vi "4.vi"() -> ()   [LabVIEW 2017]
panel:
  out "XY图":cluster{dbl[], dbl[]}[](graph)
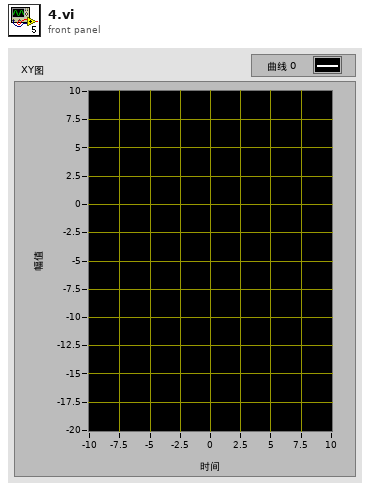
[diagram p1: front panel]
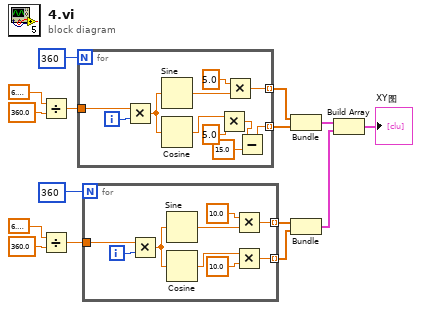
[diagram p0: block diagram]
diagram:
  n1 = Divide(x=6.283185307179586, y=360.0) -> (x/y=w12:dbl)
  n2 = Divide(x=6.283185307179586, y=360.0) -> (x/y=w6:dbl)
  n3 = for {
    N: 360 -> [_]
    tunnel: w12 -> [w26]
    tunnel: [w19] -> w11 mode=indexing
    tunnel: [w18] -> w10 mode=indexing
    i -> [w25]
    n4 = Multiply(x=w26, y=w25) -> (x*y=w24:dbl)
    n5 = Sine(x=w24) -> (sin(x)=w23:dbl)
    n6 = Cosine(x=w24) -> (cos(x)=w22:dbl)
    n7 = Multiply(x=w22, y=5.0) -> (x*y=w17:dbl)
    n8 = Multiply(x=5.0, y=w23) -> (x*y=w19:dbl)
    n9 = Subtract(x=w17, y=15.0) -> (x-y=w18:dbl)
  }
  n10 = for {
    N: 360 -> [_]
    tunnel: w6 -> [w35]
    tunnel: [w28] -> w5 mode=indexing
    tunnel: [w27] -> w4 mode=indexing
    i -> [w34]
    n11 = Multiply(x=w35, y=w34) -> (x*y=w33:dbl)
    n12 = Sine(x=w33) -> (sin(x)=w32:dbl)
    n13 = Cosine(x=w33) -> (cos(x)=w31:dbl)
    n14 = Multiply(x=10.0, y=w32) -> (x*y=w28:dbl)
    n15 = Multiply(x=w31, y=10.0) -> (x*y=w27:dbl)
  }
  n16 = Bundle(w11, w10) -> (w3:cluster{dbl[], dbl[]})  [unwired: 1 in]
  n17 = Bundle(w5, w4) -> (w2:cluster{dbl[], dbl[]})  [unwired: 1 in]
  n18 = Build Array(w3, w2) -> (→"XY图":cluster{dbl[], dbl[]}[])
